vi "Compile - Tx Packet Information.vi"(8 "error in (no error)":errorcluster, 11 "Custom Device Ref in":T1 format="%.0x") -> (0 "error out":errorcluster, 1 "Tx Ref Array":T2(array[cluster]) {"VS Refs" format="%.0x"}, 2 "Tx Packet Info Array":T3[](array[typedef]) {"targetPriority" min=1 step=1; "targetProcessor" min=-2 max=16 step=1; "Endianness" items=["big-endian"=0, "little-indian"=2]}, 3 "Custom Device Ref out":T1 format="%.0x")   [LabVIEW 2019, in "UDP-Custom-Device System Explorer.lvlib"]
uses:
  UDP-Custom-Device System Explorer.lvlib
  Shared/Types/Shared - Tx.PacketInfo.ctl
  Shared/Types/Shared - Transmit Flag Options.ctl
  Shared/Types/Shared - Transmit Echo Options.ctl
  Shared/Types/Shared - Transmit Sim Options.ctl
  Shared/Types/Shared - Channel Data Type.ctl
  Shared/Types/Shared - Header Details.ctl
  Shared/Types/Shared - Buffered.PacketInfo.ctl
  Shared/Types/Shared - Pointer Encoding.ctl
  Shared/Types/Shared - Receive Buffer Options.ctl
  Shared/Types/Shared - Transmit Buffer Options.ctl
  Shared/Types/Shared - Duplex Settings.ctl
  Shared/Types/Shared - Thread Management.ctl
  <vilib>/NI VeriStand/Custom Device API/Custom Device Item Ref.ctl
  Types/Threading/Thread Sync Reference.ctl
  Shared/UDP-Custom-Device Shared.lvlib
  <vilib>/NI VeriStand/Custom Device API/Custom Device API.lvlib
  Property Accessors/Tx Packet Accessors.lvlib
  Property Accessors/Shared Packet Accessors.lvlib
  Property Accessors/Buffered Data Packet.lvlib
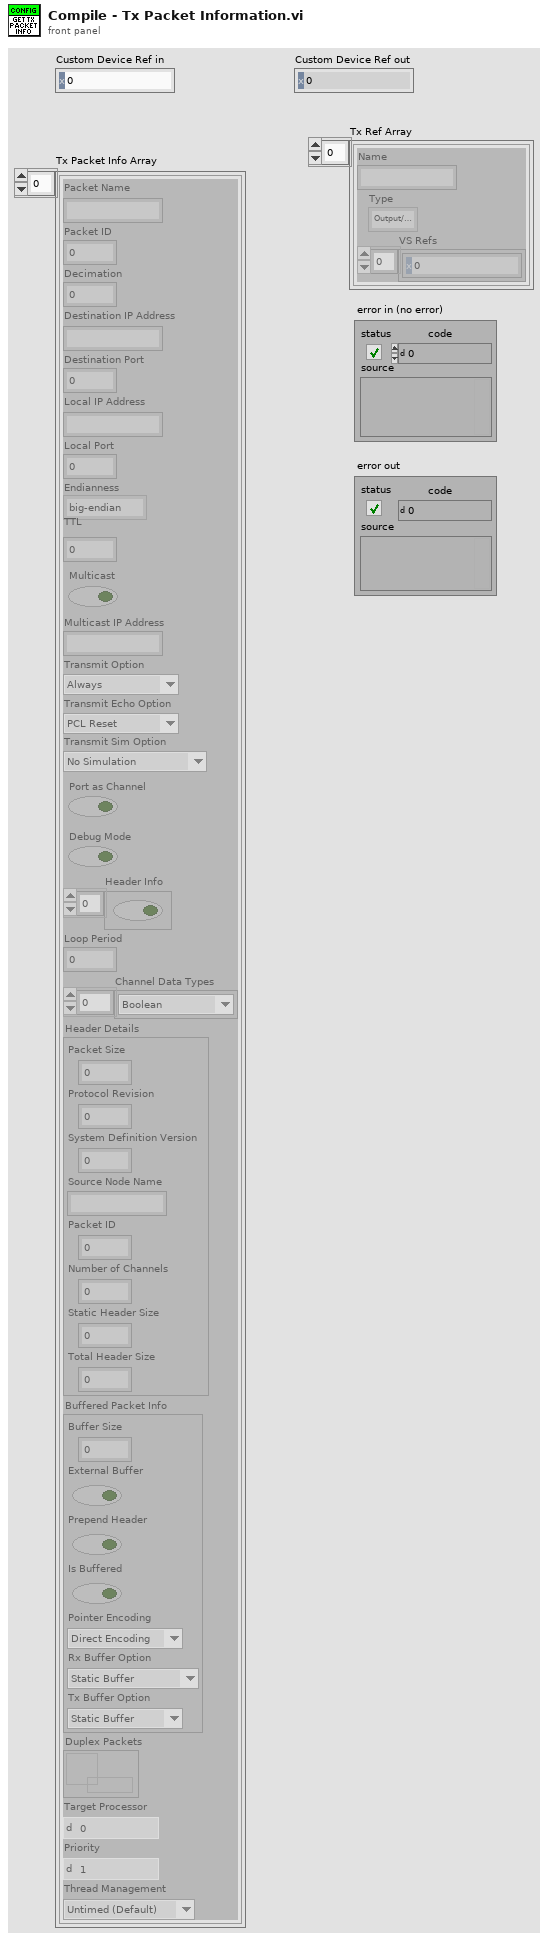
[diagram p1: front panel]
types:
  T1 = typedef "Custom Device API.lvlib/Custom Device Item Ref.ctl" = u64
  T2 = cluster{"Name":string, "Type":enum16{"Output/Write", "Input/Read", "Input/ReadWrite"}, "VS Refs":T1[]}[]
  T3 = typedef "UDP-Custom-Device Shared.lvlib/Shared - Tx.PacketInfo.ctl" = cluster{"Packet Name":string, "Packet ID":i32, "Decimation":u16, "Destination IP Address":string, "Destination Port":u16, "Local IP Address":string, "Local Port":u16, "Endianness":u16, "TTL":u16, "Multicast":bool, "Multicast IP Address":string, "Transmit Option":T4, "Transmit Echo Option":T5, "Transmit Sim Option":T6, "Port as Channel":bool, "Debug Mode":bool, "Header Info":bool[], "Loop Period":u32, "Channel Data Types":T7[], "Header Details":T8, "Buffered Packet Info":T9, "Duplex Packets":refnum<data-value>, "targetProcessor":i8, "targetPriority":i16, "Thread Management":T13}
  T4 = typedef "UDP-Custom-Device Shared.lvlib/Shared - Transmit Flag Options.ctl" = enum16{"Always", "One-Shot", "Toggle"}
  T5 = typedef "UDP-Custom-Device Shared.lvlib/Shared - Transmit Echo Options.ctl" = enum16{"PCL Reset", "Counter", "Mirror"}
  T6 = typedef "UDP-Custom-Device Shared.lvlib/Shared - Transmit Sim Options.ctl" = enum16{"No Simulation", "Counter", "Full Buffer", "FIFO Test", "FIFO + Port Test"}
  T7 = typedef "UDP-Custom-Device Shared.lvlib/Shared - Channel Data Type.ctl" = enum16{"Boolean", "Single", "Double", "I8", "I16", "I32", "I64", "U8", "U16", "U32", "U64"}
  T8 = typedef "UDP-Custom-Device Shared.lvlib/Shared - Header Details.ctl" = cluster{"Packet Size":u16, "Protocol Revision":u8, "System Definition Version":u64, "Source Node Name":string, "Packet ID":u32, "Number of Channels":u32, "Static Header Size":u16, "Total Header Size":u16}
  T9 = typedef "UDP-Custom-Device Shared.lvlib/Shared - Buffered.PacketInfo.ctl" = cluster{"Buffer Size":i32, "External Buffer":bool, "Prepend Header":bool, "Is Buffered":bool, "Pointer Encoding":T10, "Rx Buffer Option":T11, "Tx Buffer Option":T12}
  T10 = typedef "UDP-Custom-Device Shared.lvlib/Shared - Pointer Encoding.ctl" = enum16{"Direct Encoding", "Conversion Encoding"}
  T11 = typedef "UDP-Custom-Device Shared.lvlib/Shared - Receive Buffer Options.ctl" = enum16{"Static Buffer", "Circular Buffer", "Circular Buffer + Size", "Internal Cache", "Internal Cache + Size", "Ping Pong", "Ping Pong + Size"}
  T12 = typedef "UDP-Custom-Device Shared.lvlib/Shared - Transmit Buffer Options.ctl" = enum16{"Static Buffer", "FIFO Buffer", "FIFO Buffer + Port"}
  T13 = typedef "UDP-Custom-Device Shared.lvlib/Shared - Thread Management.ctl" = enum16{"Untimed (Default)", "Timed (High Priority)"}
  T14 = typedef "UDP-Custom-Device System Explorer.lvlib/Thread Sync Reference.ctl" = enum16{"PCL", "Async"}
  T15 = typedef "UDP-Custom-Device System Explorer.lvlib/Packet Type.ctl" = enum16{"Transmit", "Receive", "Buffered Transmit", "Buffered Receive"}
  T16 = typedef "Custom Device API.lvlib/Custom Device Item Info.ctl" = cluster{"Name":string, "Is Channel":bool, "GUID":string, "Is Waveform":bool}
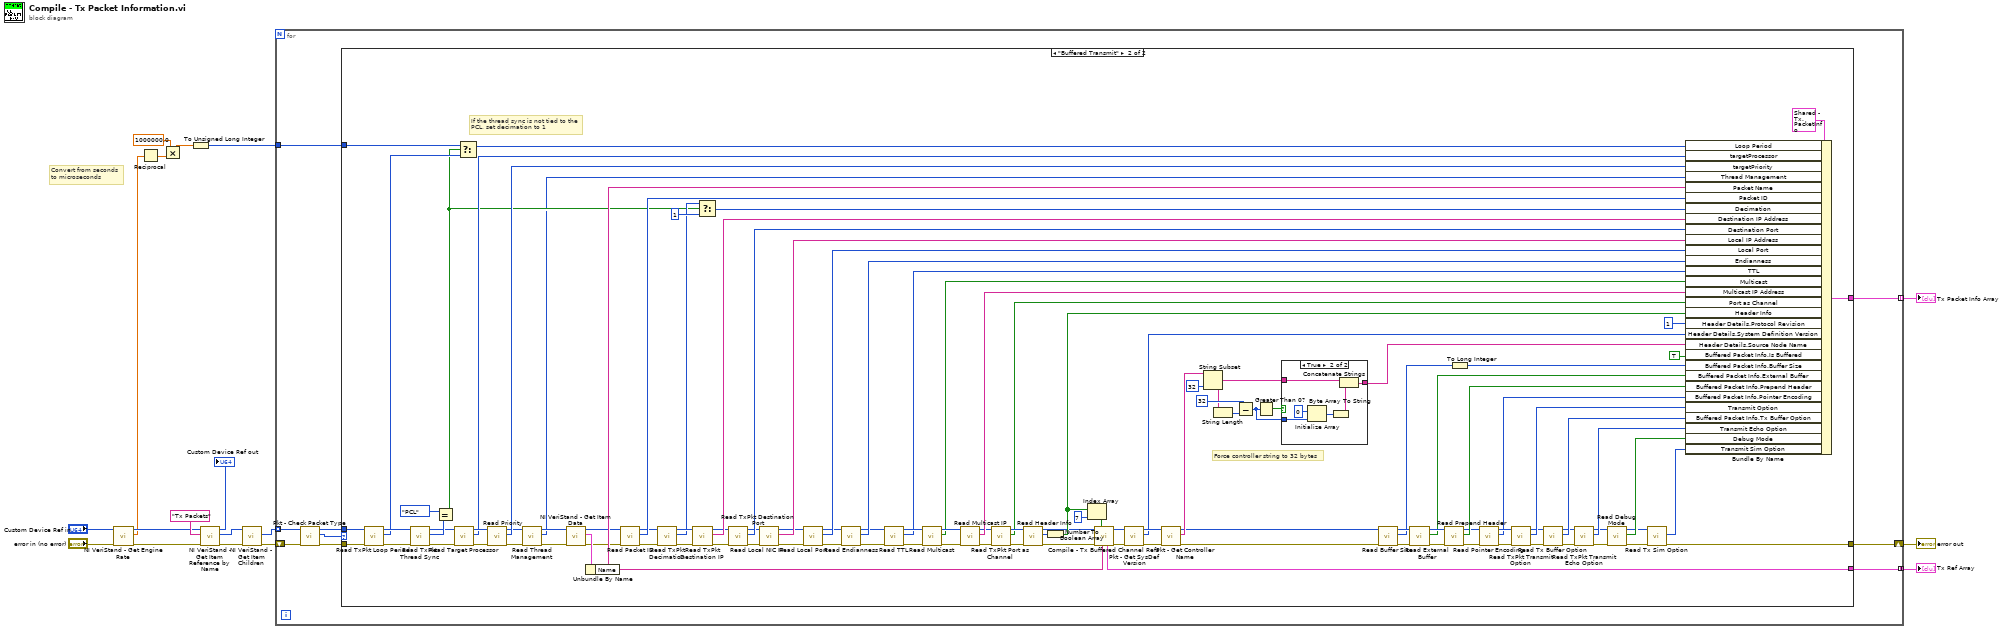
[diagram p0: block diagram]
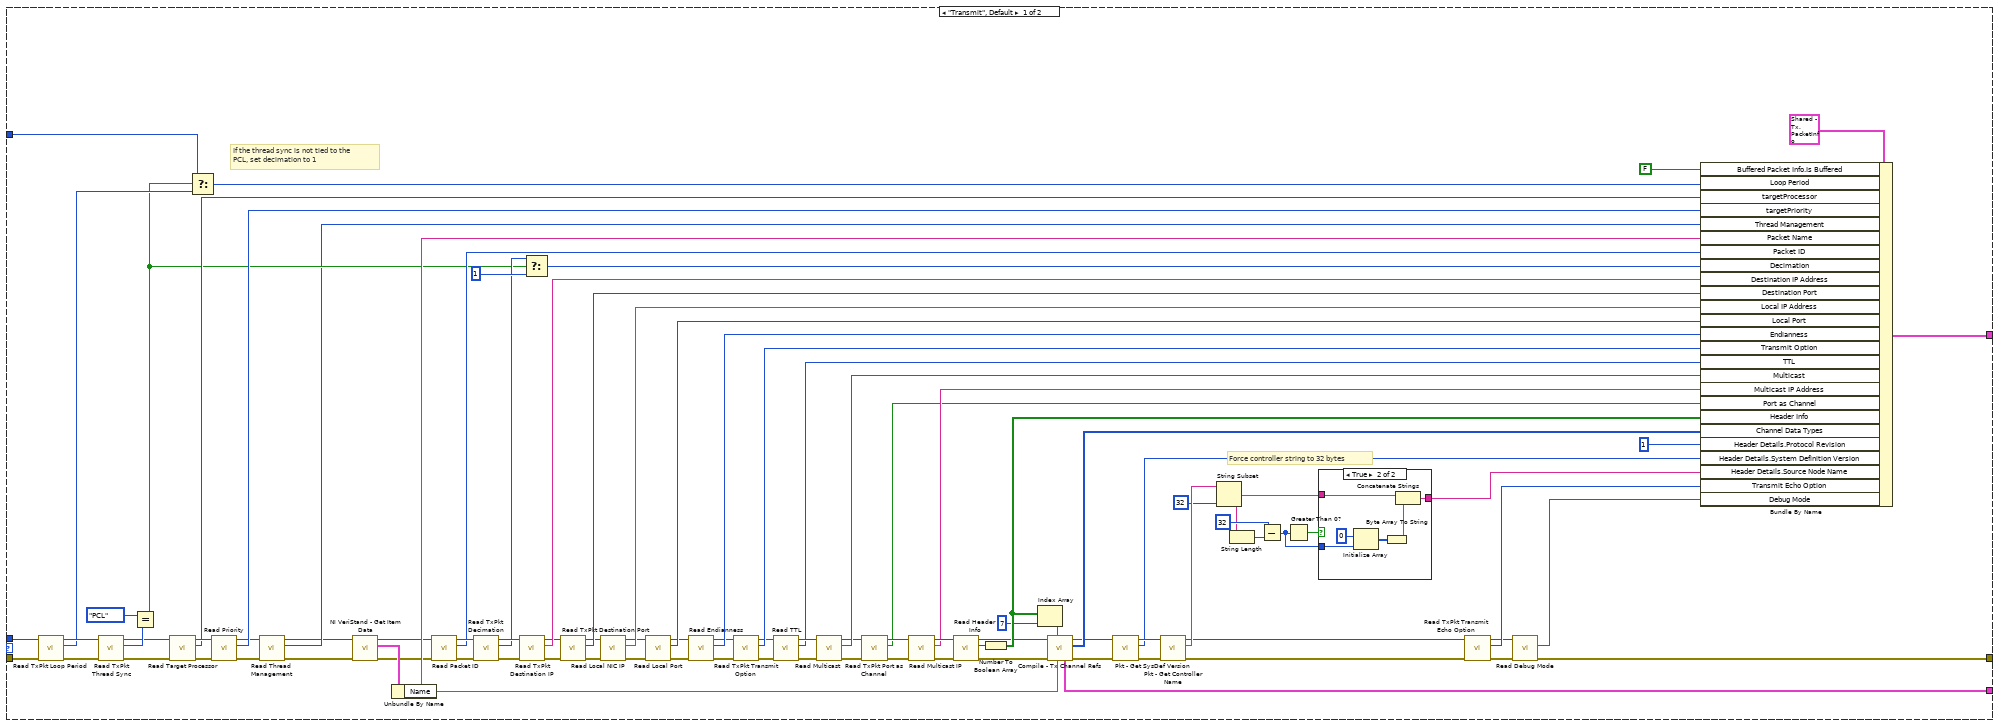
[diagram p2: hidden frame]
diagram:
  # "Convert from seconds\nto microseconds"
  n1 = call <vilib>:"NI VeriStand - Get Engine Rate.vi"("error in (no error)"="error in (no error)", "Item Ref in"="Custom Device Ref in") -> ("error out"=w7:errorcluster, "Rate (Hz)"=w5:dbl, "Item Ref out"=w6:T1)  [unwired: 7 in]
  n2 = Reciprocal(x=w5) -> (1/x=w1:dbl)
  n3 = Multiply(x=1000000.0, y=w1) -> (x*y=w3:dbl)
  n4 = To Unsigned Long Integer(number=w3) -> (unsigned 32bit integer=w4:u32)
  n5 = call <vilib>:"NI VeriStand - Get Item Reference by Name.vi"("error in (no error)"=w7, "Item Name"="Tx Packets", "Parent Ref in"=w6) -> ("error out"=w13:errorcluster, "Item Ref"=w11:T1, "Parent Ref out"=→"Custom Device Ref out":T1)  [unwired: 5 in, 1 out]
  n6 = call <vilib>:"NI VeriStand - Get Item Children.vi"("error in (no error)"=w13, "Item Ref in"=w11) -> ("error out"=w16:errorcluster, "Child Refs"=w15:T1[])  [unwired: 6 in, 2 out]
  n7 = for {
    shift-right: [w24] -> w18
    shift-left: w16 -> [w23]
    tunnel: [w27] -> w17 mode=indexing
    tunnel: w15 -> [w21] mode=indexing
    tunnel: [w25] -> w14 mode=concatenating
    tunnel: w4 -> [w26]
    n8 = call "Pkt - Check Packet Type.vi"("error in (no error)"=w23, "Node Ptr In"=w21) -> ("error out"=w22:errorcluster, "Packet Type"=w19:T15, "Node Ptr Out"=w20:T1)  [unwired: 7 in]
    n9 = case shown="\"Buffered Transmit\"" w19 {
      tunnel: [w121 w242] -> w27
      tunnel: w26 -> [w39 w147]
      tunnel: [w87 w199] -> w25
      tunnel: [w64 w166] -> w24
      tunnel: w20 -> [w43 w152]
      tunnel: w22 -> [w45 w153]
      frame "Transmit", Default {
        # "If the thread sync is not tied to the\nPCL, set decimation to 1"
        # "Force controller string to 32 bytes"
        n10 = call "Read TxPkt Loop Period.vi"("error in (no error)"=w45, "Node Ptr"=w43) -> ("error out"=w51:errorcluster, "loopPeriod"=w40:u32, "Node Ptr out"=w52:T1)  [unwired: 7 in]
        n11 = call "Read TxPkt Thread Sync.vi"("error in (no error)"=w51, "Node Ptr"=w52) -> ("error out"=w46:errorcluster, "threadSync"=w50:T14, "Node Ptr out"=w44:T1)  [unwired: 7 in]
        n12 = Equal?(x=Thread_Sync_Reference."PCL", y=w50) -> (x = y?=w33:bool)
        n13 = call "Read Target Processor.vi"("error in (no error)"=w46, "Node Ptr"=w44) -> ("error out"=w47:errorcluster, "targetProcessor"=w42:i8, "Node Ptr out"=w48:T1)  [unwired: 7 in]
        n14 = Select(t=w39, s=w33, f=w40) -> (s? t:f=w38:u32)
        n15 = call "Read Priority.vi"("error in (no error)"=w47, "Node Ptr"=w48) -> ("error out"=w31:errorcluster, "targetPriority"=w41:i16, "Node Ptr out"=w29:T1)  [unwired: 7 in]
        n16 = call "Read Thread Management.vi"("error in (no error)"=w31, "Node Ptr"=w29) -> ("error out"=w30:errorcluster, "Thread Management"=w32:T13, "Node Ptr out"=w28:T1)  [unwired: 7 in]
        n17 = call <vilib>:"NI VeriStand - Get Item Data.vi"("error in (no error)"=w30, "Item Ref in"=w28) -> ("error out"=w53:errorcluster, "Item Info"=w90:T16, "Item Ref out"=w54:T1)  [unwired: 6 in, 1 out]
        n18 = Unbundle By Name(w90) -> ("Name"=w89:string)
        n19 = call "Read Packet ID.vi"("error in (no error)"=w53, "Node Ptr"=w54) -> ("error out"=w57:errorcluster, "Packet ID"=w37:i32, "Node Ptr out"=w58:T1)  [unwired: 7 in]
        n20 = call "Read TxPkt Decimation.vi"("error in (no error)"=w57, "Node Ptr"=w58) -> ("error out"=w55:errorcluster, "Decimation"=w35:u16, "Node Ptr out"=w56:T1)  [unwired: 7 in]
        n21 = call "Read TxPkt Destination IP.vi"("error in (no error)"=w55, "Node Ptr"=w56) -> ("error out"=w59:errorcluster, "Destination IP"=w101:string, "Node Ptr out"=w60:T1)  [unwired: 7 in]
        n22 = Select(t=w35, s=w33, f=u16 1) -> (s? t:f=w34:u16)
        n23 = call "Read TxPkt Destination Port.vi"("error in (no error)"=w59, "Node Ptr"=w60) -> ("error out"=w61:errorcluster, "Destination Port"=w102:u16, "Node Ptr out"=w62:T1)  [unwired: 7 in]
        n24 = call "Read Local NIC IP.vi"("error in (no error)"=w61, "Node Ptr"=w62) -> ("error out"=w98:errorcluster, "IP Address of Local NIC"=w100:string, "Node Ptr out"=w99:T1)  [unwired: 7 in]
        n25 = call "Read Local Port.vi"("error in (no error)"=w98, "Node Ptr"=w99) -> ("error out"=w95:errorcluster, "Port"=w97:u16, "Node Ptr out"=w96:T1)  [unwired: 7 in]
        n26 = call "Read Endianness.vi"("error in (no error)"=w95, "Node Ptr"=w96) -> ("error out"=w86:errorcluster, "Endianness"=w94:u16, "Node Ptr out"=w85:T1)  [unwired: 7 in]
        n27 = call "Read TxPkt Transmit Option.vi"("error in (no error)"=w86, "Node Ptr"=w85) -> ("error out"=w79:errorcluster, "Transmit Options"=w84:T4, "Node Ptr out"=w81:T1)  [unwired: 7 in]
        n28 = call "Read TTL.vi"("error in (no error)"=w79, "Node Ptr"=w81) -> ("error out"=w83:errorcluster, "TTL"=w77:u16, "Node Ptr out"=w82:T1)  [unwired: 7 in]
        n29 = call "Read Multicast.vi"("error in (no error)"=w83, "Node Ptr"=w82) -> ("error out"=w72:errorcluster, "Multicast"=w76:bool, "Node Ptr out"=w74:T1)  [unwired: 7 in]
        n30 = call "Read TxPkt Port as Channel.vi"("error in (no error)"=w72, "Node Ptr"=w74) -> ("error out"=w71:errorcluster, "Port as Channel"=w70:bool, "Node Ptr out"=w73:T1)  [unwired: 7 in]
        n31 = call "Read Multicast IP.vi"("error in (no error)"=w71, "Node Ptr"=w73) -> ("error out"=w78:errorcluster, "Multicast IP Address"=w75:string, "Node Ptr out"=w80:T1)  [unwired: 7 in]
        n32 = call "Read Header Info.vi"("error in (no error)"=w78, "Node Ptr"=w80) -> ("error out"=w91:errorcluster, "Header Info"=w92:u32, "Node Ptr out"=w93:T1)  [unwired: 7 in]
        n33 = Number To Boolean Array(number=w92) -> (Boolean array=w119:bool[])
        n34 = Index Array(array=w119, index=7) -> (element=w117:bool)
        n35 = call "Compile - Tx Channel Refs.vi"("Packet Name"=w89, "Timestamp Present?"=w117, "error in (no error)"=w91, "Item Ref in"=w93) -> ("error out"=w105:errorcluster, "Data types"=w116:T7[], "Item Ref out"=w107:T1, "Tx Ref Array"=w87:T2)  [unwired: 4 in]
        n36 = call "Pkt - Get SysDef Version.vi"("error in (no error)"=w105, "Packet Ref In"=w107) -> ("error out"=w104:errorcluster, "Encoded Version"=w103:u64, "Packet Ref out"=w106:T1)  [unwired: 6 in, 1 out]
        n37 = call "Pkt - Get Controller Name.vi"("error in (no error)"=w104, "Packet Ref In"=w106) -> ("error out"=w68:errorcluster, "Name"=w115:string, "Packet Ref out"=w69:T1)  [unwired: 7 in]
        n38 = String Subset(string=w115, length (rest)=32 ("length (rest)")) -> (substring=w109:string)  [unwired: 1 in]
        n39 = String Length(string=w109) -> (length=w112:i32)
        n40 = Subtract(x=32 ("length (rest)"), y=w112) -> (x-y=w110:i32)
        n41 = Greater Than 0?(x=w110) -> (x > 0?=w111:bool)
        n42 = case shown="True" w111 {
          tunnel: w110 -> [_ w129]
          tunnel: w109 -> [w123 w126]
          tunnel: [w123 w124] -> w108
          frame False {
          }
          frame True {
            n43 = Initialize Array(u8 0, w129) -> (w127:u8[])
            n44 = Byte Array To String(unsigned byte array=w127) -> (string=w125:string)
            n45 = Concatenate Strings(w126, w125) -> (w124:string)
          }
        }
        n46 = call "Read TxPkt Transmit Echo Option.vi"("error in (no error)"=w68, "Node Ptr"=w69) -> ("error out"=w65:errorcluster, "Transmit Echo Options"=w67:T5, "Node Ptr out"=w66:T1)  [unwired: 7 in]
        n47 = call "Read Debug Mode.vi"("error in (no error)"=w65, "Node Ptr"=w66) -> ("error out"=w64:errorcluster, "Debug Mode"=w63:bool)  [unwired: 7 in, 1 out]
        n48 = Bundle By Name(cluster=T3 {"Packet Name"="", "Packet ID"=0, "Decimation"=0, "Destination IP Address"="", "Destination Port"=0, "Local IP Address"="", "Local Port"=0, "Endianness"=0, "TTL"=0, "Multicast"=FALSE, "Multicast IP Address"="", "Transmit Option"=enum."Always", "Transmit Echo Option"=enum."PCL Reset", "Transmit Sim Option"=enum."No Simulation", "Port as Channel"=FALSE, "Debug Mode"=FALSE, "Header Info"=[], "Loop Period"=0, "Channel Data Types"=[], "Header Details"={"Packet Size"=0, "Protocol Revision"=0, "System Definition Version"=0, "Source Node Name"="", "Packet ID"=0, "Number of Channels"=0, "Static Header Size"=0, "Total Header Size"=0}, "Buffered Packet Info"={"Buffer Size"=0, "External Buffer"=FALSE, "Prepend Header"=FALSE, "Is Buffered"=FALSE, "Pointer Encoding"=enum."Direct Encoding", "Rx Buffer Option"=enum."Static Buffer", "Tx Buffer Option"=enum."Static Buffer"}, "Duplex Packets"=refnum, "targetProcessor"=0, "targetPriority"=1, "Thread Management"=enum."Untimed (Default)"} ("Packet Info"), "Buffered Packet Info.Is Buffered"=FALSE, "Loop Period"=w38, "targetProcessor"=w42, "targetPriority"=w41, "Thread Management"=w32, "Packet Name"=w89, "Packet ID"=w37, "Decimation"=w34, "Destination IP Address"=w101, "Destination Port"=w102, "Local IP Address"=w100, "Local Port"=w97, "Endianness"=w94, "Transmit Option"=w84, "TTL"=w77, "Multicast"=w76, "Multicast IP Address"=w75, "Port as Channel"=w70, "Header Info"=w119, "Channel Data Types"=w116, "Header Details.Protocol Revision"=u8 1, "Header Details.System Definition Version"=w103, "Header Details.Source Node Name"=w108, "Transmit Echo Option"=w67, "Debug Mode"=w63) -> (w121:T3)
      }
      frame "Buffered Transmit" {
        # "If the thread sync is not tied to the\nPCL, set decimation to 1"
        # "Force controller string to 32 bytes"
        n49 = call "Read TxPkt Loop Period.vi"("error in (no error)"=w153, "Node Ptr"=w152) -> ("error out"=w150:errorcluster, "loopPeriod"=w145:u32, "Node Ptr out"=w151:T1)  [unwired: 7 in]
        n50 = call "Read TxPkt Thread Sync.vi"("error in (no error)"=w150, "Node Ptr"=w151) -> ("error out"=w141:errorcluster, "threadSync"=w149:T14, "Node Ptr out"=w143:T1)  [unwired: 7 in]
        n51 = Equal?(x=Thread_Sync_Reference."PCL", y=w149) -> (x = y?=w135:bool)
        n52 = call "Read Target Processor.vi"("error in (no error)"=w141, "Node Ptr"=w143) -> ("error out"=w142:errorcluster, "targetProcessor"=w140:i8, "Node Ptr out"=w144:T1)  [unwired: 7 in]
        n53 = Select(t=w147, s=w135, f=w145) -> (s? t:f=w146:u32)
        n54 = call "Read Priority.vi"("error in (no error)"=w142, "Node Ptr"=w144) -> ("error out"=w132:errorcluster, "targetPriority"=w139:i16, "Node Ptr out"=w134:T1)  [unwired: 7 in]
        n55 = call "Read Thread Management.vi"("error in (no error)"=w132, "Node Ptr"=w134) -> ("error out"=w131:errorcluster, "Thread Management"=w130:T13, "Node Ptr out"=w133:T1)  [unwired: 7 in]
        n56 = call <vilib>:"NI VeriStand - Get Item Data.vi"("error in (no error)"=w131, "Item Ref in"=w133) -> ("error out"=w155:errorcluster, "Item Info"=w216:T16, "Item Ref out"=w156:T1)  [unwired: 6 in, 1 out]
        n57 = Unbundle By Name(w216) -> ("Name"=w200:string)
        n58 = call "Read Packet ID.vi"("error in (no error)"=w155, "Node Ptr"=w156) -> ("error out"=w157:errorcluster, "Packet ID"=w225:i32, "Node Ptr out"=w158:T1)  [unwired: 7 in]
        n59 = call "Read TxPkt Decimation.vi"("error in (no error)"=w157, "Node Ptr"=w158) -> ("error out"=w159:errorcluster, "Decimation"=w137:u16, "Node Ptr out"=w160:T1)  [unwired: 7 in]
        n60 = call "Read TxPkt Destination IP.vi"("error in (no error)"=w159, "Node Ptr"=w160) -> ("error out"=w162:errorcluster, "Destination IP"=w226:string, "Node Ptr out"=w163:T1)  [unwired: 7 in]
        n61 = Select(t=w137, s=w135, f=u16 1) -> (s? t:f=w136:u16)
        n62 = call "Read TxPkt Destination Port.vi"("error in (no error)"=w162, "Node Ptr"=w163) -> ("error out"=w161:errorcluster, "Destination Port"=w227:u16, "Node Ptr out"=w164:T1)  [unwired: 7 in]
        n63 = call "Read Local NIC IP.vi"("error in (no error)"=w161, "Node Ptr"=w164) -> ("error out"=w222:errorcluster, "IP Address of Local NIC"=w224:string, "Node Ptr out"=w223:T1)  [unwired: 7 in]
        n64 = call "Read Local Port.vi"("error in (no error)"=w222, "Node Ptr"=w223) -> ("error out"=w219:errorcluster, "Port"=w221:u16, "Node Ptr out"=w220:T1)  [unwired: 7 in]
        n65 = call "Read Endianness.vi"("error in (no error)"=w219, "Node Ptr"=w220) -> ("error out"=w191:errorcluster, "Endianness"=w218:u16, "Node Ptr out"=w192:T1)  [unwired: 7 in]
        n66 = call "Read TTL.vi"("error in (no error)"=w191, "Node Ptr"=w192) -> ("error out"=w195:errorcluster, "TTL"=w190:u16, "Node Ptr out"=w194:T1)  [unwired: 7 in]
        n67 = call "Read Multicast.vi"("error in (no error)"=w195, "Node Ptr"=w194) -> ("error out"=w196:errorcluster, "Multicast"=w189:bool, "Node Ptr out"=w193:T1)  [unwired: 7 in]
        n68 = call "Read Multicast IP.vi"("error in (no error)"=w196, "Node Ptr"=w193) -> ("error out"=w182:errorcluster, "Multicast IP Address"=w188:string, "Node Ptr out"=w180:T1)  [unwired: 7 in]
        n69 = call "Read TxPkt Port as Channel.vi"("error in (no error)"=w182, "Node Ptr"=w180) -> ("error out"=w181:errorcluster, "Port as Channel"=w178:bool, "Node Ptr out"=w179:T1)  [unwired: 7 in]
        n70 = call "Read Header Info.vi"("error in (no error)"=w181, "Node Ptr"=w179) -> ("error out"=w203:errorcluster, "Header Info"=w217:u32, "Node Ptr out"=w204:T1)  [unwired: 7 in]
        n71 = Number To Boolean Array(number=w217) -> (Boolean array=w240:bool[])
        n72 = Index Array(array=w240, index=7) -> (element=w205:bool)
        n73 = call "Compile - Tx Buffered Channel Refs.vi"("Packet Name"=w200, "Timestamp Present?"=w205, "error in (no error)"=w203, "Item Ref in"=w204) -> ("error out"=w201:errorcluster, "Item Ref out"=w202:T1, "Tx Ref Array"=w199:T2)  [unwired: 5 in]
        n74 = call "Pkt - Get SysDef Version.vi"("error in (no error)"=w201, "Packet Ref In"=w202) -> ("error out"=w229:errorcluster, "Encoded Version"=w228:u64, "Packet Ref out"=w230:T1)  [unwired: 6 in, 1 out]
        n75 = call "Pkt - Get Controller Name.vi"("error in (no error)"=w229, "Packet Ref In"=w230) -> ("error out"=w209:errorcluster, "Name"=w238:string, "Packet Ref out"=w214:T1)  [unwired: 7 in]
        n76 = String Subset(string=w238, length (rest)=32 ("length (rest)")) -> (substring=w232:string)  [unwired: 1 in]
        n77 = String Length(string=w232) -> (length=w235:i32)
        n78 = Subtract(x=32 ("length (rest)"), y=w235) -> (x-y=w233:i32)
        n79 = Greater Than 0?(x=w233) -> (x > 0?=w234:bool)
        n80 = case shown="True" w234 {
          tunnel: w233 -> [_ w249]
          tunnel: w232 -> [w243 w246]
          tunnel: [w243 w244] -> w231
          frame False {
          }
          frame True {
            n81 = Initialize Array(u8 0, w249) -> (w247:u8[])
            n82 = Byte Array To String(unsigned byte array=w247) -> (string=w245:string)
            n83 = Concatenate Strings(w246, w245) -> (w244:string)
          }
        }
        n84 = call "Read Buffer Size.vi"("error in (no error)"=w209, "Node Ptr"=w214) -> ("error out"=w211:errorcluster, "Buffer Size"=w208:u32, "Node Ptr out"=w213:T1)  [unwired: 7 in]
        n85 = call "Read External Buffer.vi"("error in (no error)"=w211, "Node Ptr"=w213) -> ("error out"=w210:errorcluster, "External Buffer"=w207:bool, "Node Ptr out"=w212:T1)  [unwired: 7 in]
        n86 = call "Read Prepend Header.vi"("error in (no error)"=w210, "Node Ptr"=w212) -> ("error out"=w185:errorcluster, "Prepend Header"=w206:bool, "Node Ptr out"=w187:T1)  [unwired: 7 in]
        n87 = To Long Integer(number=w208) -> (32bit integer=w198:i32)
        n88 = call "Read Pointer Encoding.vi"("error in (no error)"=w185, "Node Ptr"=w187) -> ("error out"=w184:errorcluster, "Pointer Encoding"=w183:T10, "Node Ptr out"=w186:T1)  [unwired: 7 in]
        n89 = call "Read TxPkt Transmit Option.vi"("error in (no error)"=w184, "Node Ptr"=w186) -> ("error out"=w176:errorcluster, "Transmit Options"=w197:T4, "Node Ptr out"=w177:T1)  [unwired: 7 in]
        n90 = call "Read Tx Buffer Option.vi"("error in (no error)"=w176, "Node Ptr"=w177) -> ("error out"=w173:errorcluster, "Buffer Option"=w175:T12, "Node Ptr out"=w174:T1)  [unwired: 7 in]
        n91 = call "Read TxPkt Transmit Echo Option.vi"("error in (no error)"=w173, "Node Ptr"=w174) -> ("error out"=w170:errorcluster, "Transmit Echo Options"=w172:T5, "Node Ptr out"=w171:T1)  [unwired: 7 in]
        n92 = call "Read Debug Mode.vi"("error in (no error)"=w170, "Node Ptr"=w171) -> ("error out"=w167:errorcluster, "Debug Mode"=w169:bool, "Node Ptr out"=w168:T1)  [unwired: 7 in]
        n93 = call "Read Tx Sim Option.vi"("error in (no error)"=w167, "Node Ptr"=w168) -> ("error out"=w166:errorcluster, "Sim Option"=w165:T6)  [unwired: 7 in, 1 out]
        n94 = Bundle By Name(cluster=T3 {"Packet Name"="", "Packet ID"=0, "Decimation"=0, "Destination IP Address"="", "Destination Port"=0, "Local IP Address"="", "Local Port"=0, "Endianness"=0, "TTL"=0, "Multicast"=FALSE, "Multicast IP Address"="", "Transmit Option"=enum."Always", "Transmit Echo Option"=enum."PCL Reset", "Transmit Sim Option"=enum."No Simulation", "Port as Channel"=FALSE, "Debug Mode"=FALSE, "Header Info"=[], "Loop Period"=0, "Channel Data Types"=[], "Header Details"={"Packet Size"=0, "Protocol Revision"=0, "System Definition Version"=0, "Source Node Name"="", "Packet ID"=0, "Number of Channels"=0, "Static Header Size"=0, "Total Header Size"=0}, "Buffered Packet Info"={"Buffer Size"=0, "External Buffer"=FALSE, "Prepend Header"=FALSE, "Is Buffered"=FALSE, "Pointer Encoding"=enum."Direct Encoding", "Rx Buffer Option"=enum."Static Buffer", "Tx Buffer Option"=enum."Static Buffer"}, "Duplex Packets"=refnum, "targetProcessor"=0, "targetPriority"=1, "Thread Management"=enum."Untimed (Default)"} ("Packet Info"), "Loop Period"=w146, "targetProcessor"=w140, "targetPriority"=w139, "Thread Management"=w130, "Packet Name"=w200, "Packet ID"=w225, "Decimation"=w136, "Destination IP Address"=w226, "Destination Port"=w227, "Local IP Address"=w224, "Local Port"=w221, "Endianness"=w218, "TTL"=w190, "Multicast"=w189, "Multicast IP Address"=w188, "Port as Channel"=w178, "Header Info"=w240, "Header Details.Protocol Revision"=u8 1, "Header Details.System Definition Version"=w228, "Header Details.Source Node Name"=w231, "Buffered Packet Info.Is Buffered"=TRUE, "Buffered Packet Info.Buffer Size"=w198, "Buffered Packet Info.External Buffer"=w207, "Buffered Packet Info.Prepend Header"=w206, "Buffered Packet Info.Pointer Encoding"=w183, "Transmit Option"=w197, "Buffered Packet Info.Tx Buffer Option"=w175, "Transmit Echo Option"=w172, "Debug Mode"=w169, "Transmit Sim Option"=w165) -> (w242:T3)
      }
    }
  }
  "Tx Packet Info Array" <- w17
  "error out" <- w18
  "Tx Ref Array" <- w14
